vi "HoloCtrlArray.vi"(7 "Action":enum16{"READ", "WRITE"}(ring), 10 "Holo Array In":T1[](array[typedef]) {"Modes"."Amplititute" step=0.05}) -> (2 "Holo Array Out":T1[](array[typedef]) {"Modes"."Amplititute" step=0.05})   [LabVIEW 2014]
uses:
  Controls/Holo Settings.ctl
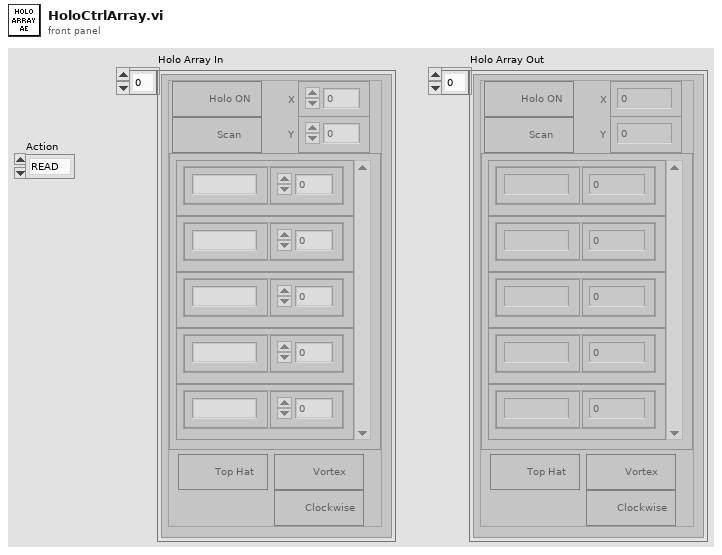
[diagram p1: front panel]
types:
  T1 = typedef "Holo Settings.ctl" = cluster{"Top Hat":bool, "Modes":cluster{"Mode ID":string, "Amplititute":dbl}[], "Vortex":bool, "Clockwise":bool, "X":dbl, "Y":dbl, "Holo ON":bool, "Scan":bool}
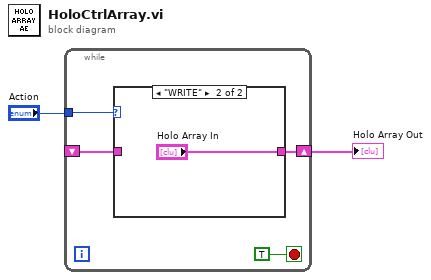
[diagram p0: block diagram]
diagram:
  n1 = while {
    shift-right: [w5] -> w1
    shift-left: _ -> [w4]
    tunnel: "Action" -> [w3]
    stop <- TRUE stop-if-true
    n2 = case shown="\"WRITE\"" w3 {
      tunnel: [w7 "Holo Array In"] -> w5
      tunnel: w4 -> [w7 _]
      frame "READ", Default {
      }
      frame "WRITE" {
      }
    }
  }
  "Holo Array Out" <- w1
